vi "test_Packet_All.vi"(8 "error in (no error)":errorcluster) -> (0 "error out":errorcluster, 3 "Test Passed":bool)   [LabVIEW 2019]
panel:
  out "SimplePipelineResult":bool
  out "SimpleTrackedTarget":bool
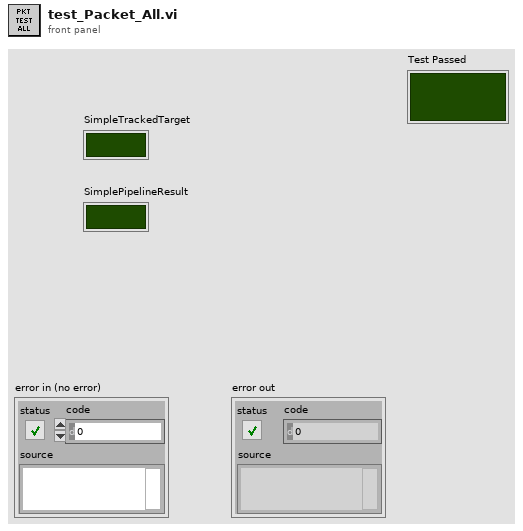
[diagram p1: front panel]
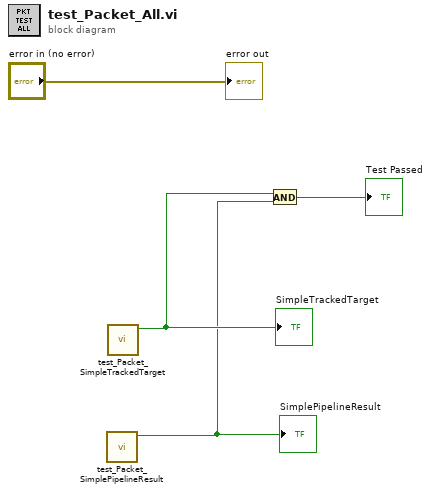
[diagram p0: block diagram]
diagram:
  n1 = call "test_Packet_SimplePipelineResult.vi"() -> ("Test Passed"=w1:bool)  [unwired: 10 in, 1 out]
  "SimplePipelineResult" <- w1
  n2 = call "test_Packet_SimpleTrackedTarget.vi"() -> ("Test Passed"=w2:bool)  [unwired: 10 in, 1 out]
  "SimpleTrackedTarget" <- w2
  n3 = And(x=w2, y=w1) -> (x .and. y?=→"Test Passed":bool)
  "error out" <- "error in (no error)"
